vi "Set Power.vi"(8 "error in (no error)":errorcluster, 9 "Power":dbl, 11 "LQ Laser Quantum in":refnum<class "LQ Laser.lvclass">) -> (0 "error out":errorcluster, 3 "LQ Laser Quantum out":refnum<class "LQ Laser.lvclass">)   [LabVIEW 2023, in "LQ Laser.lvlib" / "LQ Laser.lvclass"]
uses:
  LQ Laser.lvclass
  LQ Laser.lvclass/LQ Laser.ctl
panel:
  out "Response":string
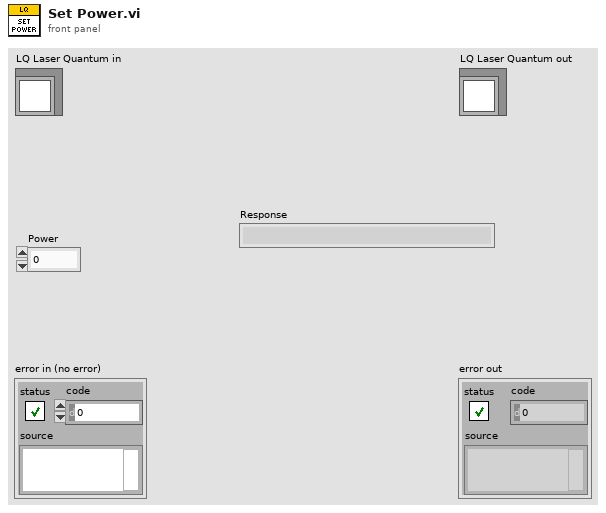
[diagram p1: front panel]
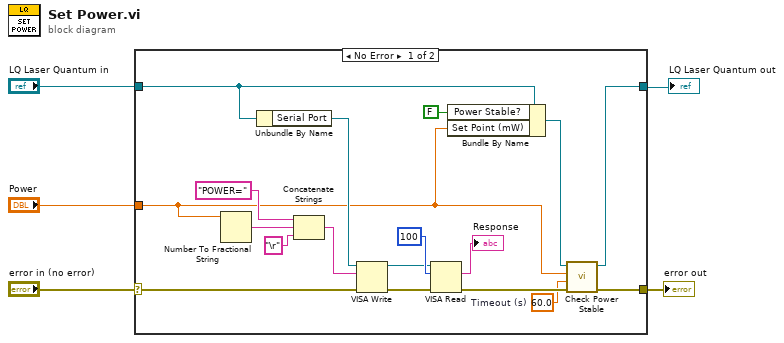
[diagram p0: block diagram]
diagram:
  n1 = case shown="No Error" "error in (no error)" {
    selector: "error in (no error)" -> [w23 w25]
    tunnel: [w11 w25] -> w1
    tunnel: "LQ Laser Quantum in" -> [w10 w24]
    tunnel: [w12 w24] -> w2
    tunnel: "Power" -> [w8 _]
    frame No Error {
      w6 = 60.0  # Timeout (s)
      n2 = Number To Fractional String(number=w8) -> (F-format string=w21:string)  [unwired: 3 in]
      n3 = Unbundle By Name(w10) -> ("Serial Port"=w18:refnum<visa-resource-name>)
      n4 = Concatenate Strings("POWER=" ("write buffer"), w21, "\r" ("string")) -> (w20:string)
      n5 = VISA Write(VISA resource name=w18, write buffer=w20, error in (no error)=w23) -> (VISA resource name out=w15:refnum<visa-resource-name>, error out=w16:errorcluster)  [unwired: 1 out]
      n6 = VISA Read(VISA resource name=w15, byte count=u32 100, error in (no error)=w16) -> (read buffer=→"Response":string, error out=w13:errorcluster)  [unwired: 2 out]
      n7 = Bundle By Name(cluster=w10, "Power Stable?"=FALSE ("Power Tuning?"), "Set Point (mW)"=w8) -> (w9:refnum<class "LQ Laser.lvclass">)
      n8 = call-dynamic "Check Power Stable.vi"("error in (no error)"=w13, "Timeout (s)"=w6, "Set Point (mW)"=w8, "LQ Laser in"=w9) -> ("error out"=w11:errorcluster, "LQ Laser out"=w12:refnum<class "LQ Laser.lvclass">)  [unwired: 6 in]
    }
    frame Error {
    }
  }
  "error out" <- w1
  "LQ Laser Quantum out" <- w2
